vi "Clear Remote CAN Logs Dir.vi"(8 "error in (no error)":errorcluster, 11 "address":string) -> (0 "error out":errorcluster, 3 "Logs To Transfer":T1[](array[typedef]))   [LabVIEW 2010, in "CAN Log Transfer and Convert.lvlib"]
uses:
  CAN Log Transfer and Convert.lvlib
  CAN Sysdef Data.ctl
  <vilib>/addons/internet/NI_InternetTK_FTP_VIs.lvlib
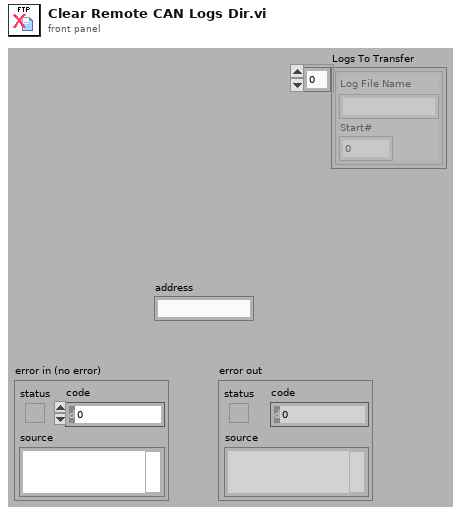
[diagram p1: front panel]
types:
  T1 = typedef "CAN Log Transfer and Convert.lvlib/CAN Sysdef Data.ctl" = cluster{"Log File Name":string, "Start#":u16}
  T2 = typedef "FTP Session.ctl" = refnum<k1>
  T3 = typedef "FTP File Info.ctl" = cluster{"type":enum16{"unknown", "file", "dir", "link"}, "permissions":string, "owner":string, "group":string, "size":i32, "date":string, "name":string, "link name":string}
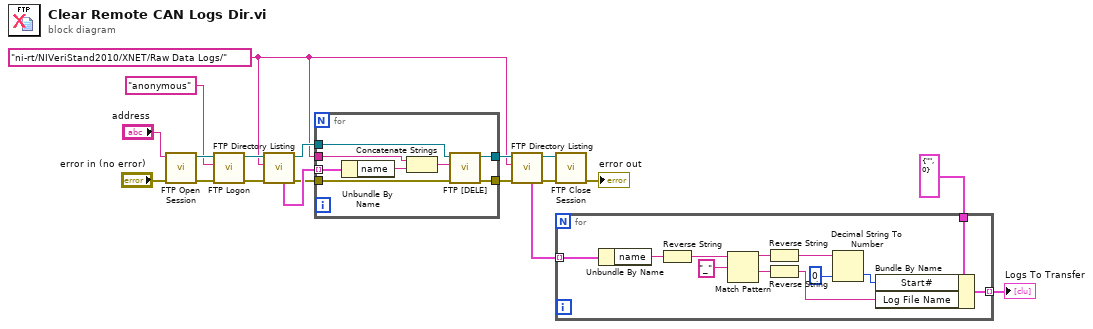
[diagram p0: block diagram]
diagram:
  w6 = "ni-rt/NIVeriStand2010/XNET/Raw Data Logs/"
  n1 = call <vilib>:"FTP Open Session.vi"("error in (no error)"="error in (no error)", "address"="address") -> ("error out"=w19:errorcluster, "ftp session"=w18:T2)  [unwired: 6 in, 2 out]
  n2 = call <vilib>:"FTP Logon.vi"("error in (no error)"=w19, "user"="anonymous", "ftp session"=w18) -> ("error out"=w13:errorcluster, "ftp session out"=w12:T2)  [unwired: 5 in, 2 out]
  n3 = call <vilib>:"FTP Directory Listing.vi"("error in (no error)"=w13, "directory path"=w6, "ftp session"=w12) -> ("error out"=w9:errorcluster, "ftp session out"=w10:T2, "dir list"=w11:T3[])  [unwired: 4 in, 2 out]
  n4 = for {
    tunnel: [w25] -> w7
    tunnel: w11 -> [w24] mode=indexing
    tunnel: w10 -> [w23]
    tunnel: w9 -> [w27]
    tunnel: [w26] -> w8
    tunnel: w6 -> [w21]
    n5 = Unbundle By Name(w24) -> ("name"=w22:string)
    n6 = Concatenate Strings(w21, w22) -> (w20:string)
    n7 = call <vilib>:"FTP [DELE].vi"("error in (no error)"=w27, "file path"=w20, "ftp session"=w23) -> ("error out"=w26:errorcluster, "ftp session out"=w25:T2)  [unwired: 5 in, 2 out]
  }
  n8 = call <vilib>:"FTP Directory Listing.vi"("error in (no error)"=w8, "directory path"=w6, "ftp session"=w7) -> ("error out"=w5:errorcluster, "ftp session out"=w4:T2, "dir list"=w3:T3[])  [unwired: 4 in, 2 out]
  n9 = call <vilib>:"FTP Close Session.vi"("error in (no error)"=w5, "ftp session"=w4) -> ("error out"=→"error out":errorcluster)  [unwired: 6 in, 3 out]
  n10 = for {
    tunnel: w3 -> [w39] mode=indexing
    tunnel: T1 {"Log File Name"="", "Start#"=0} ("CAN Sysdef") -> [w38]
    tunnel: [w37] -> w1 mode=indexing
    n11 = Unbundle By Name(w39) -> ("name"=w32:string)
    n12 = Reverse String(1:w32) -> (0:w35:string)
    n13 = Match Pattern(string=w35, regular expression="_") -> (before substring=w34:string, after substring=w30:string)  [unwired: 1 in, 2 out]
    n14 = Reverse String(1:w34) -> (0:w33:string)
    n15 = Reverse String(1:w30) -> (0:w31:string)
    n16 = Decimal String To Number(string=w33, default (0L)=u16 0) -> (number=w29:u16)  [unwired: 1 in, 1 out]
    n17 = Bundle By Name(cluster=w38, "Start#"=w29, "Log File Name"=w31) -> (w37:T1)
  }
  "Logs To Transfer" <- w1
